vi "Generate Z stage Position Aarray.vi"(7 "#rep1":i32, 8 "#rep2":u16, 9 "thickness2":dbl, 10 "Start Z":dbl format="%#_13g", 11 "thickness1":dbl) -> (3 "Array":dbl[](array[numeric]))   [LabVIEW 2018]
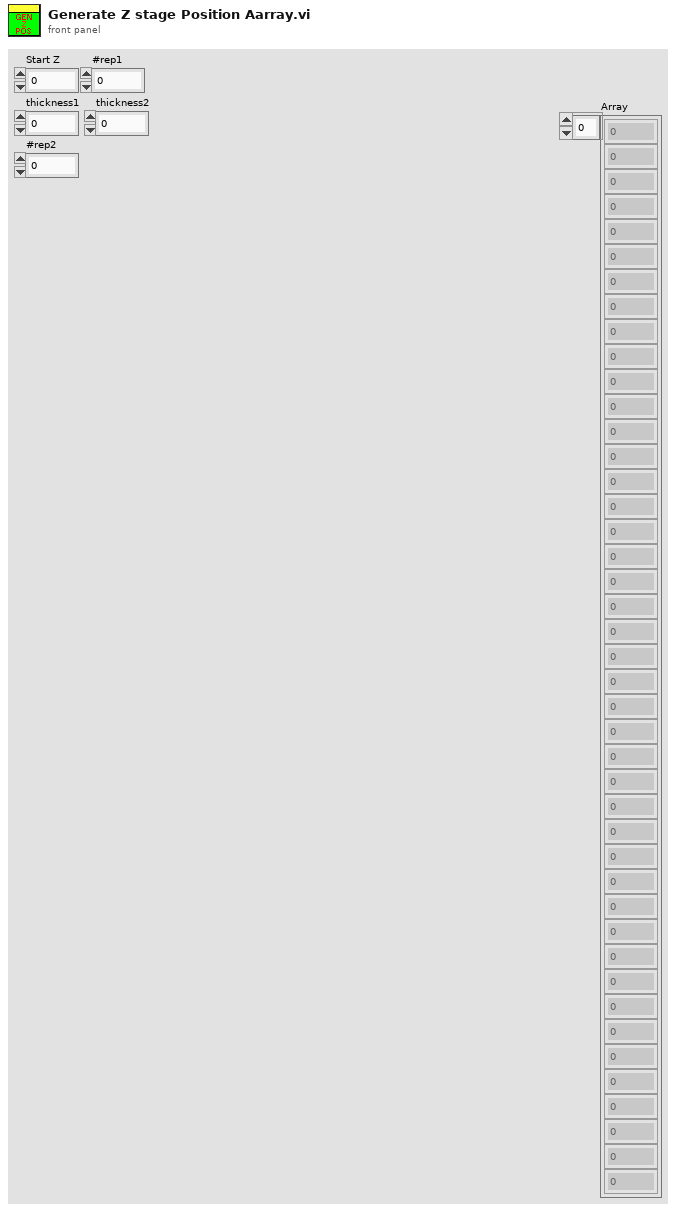
[diagram p1: front panel]
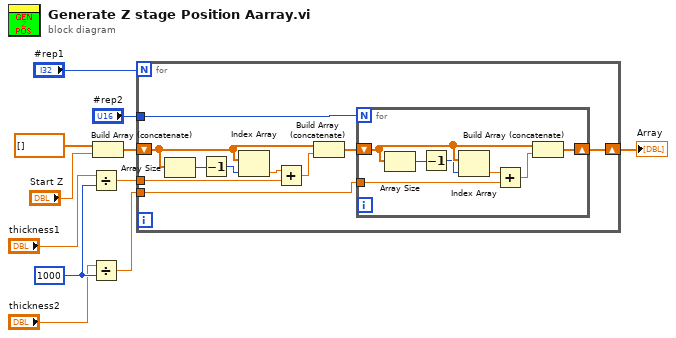
[diagram p0: block diagram]
diagram:
  w11 = 1000
  n1 = Divide(x="thickness1", y=w11) -> (x/y=w9:dbl)
  n2 = Divide(x="thickness2", y=w11) -> (x/y=w10:dbl)
  n3 = Build Array (concatenate)(dbl[] [] ("element"), "Start Z") -> (w7:dbl[])
  n4 = for {
    N: "#rep1" -> [_]
    shift-right: [w18] -> w6
    shift-left: w7 -> [w15]
    tunnel: w9 -> [w16]
    tunnel: w10 -> [w19]
    tunnel: "#rep2" -> [w21]
    n5 = Array Size(array=w15) -> (size(s)=w13:i32)
    n6 = Decrement(x=w13) -> (x-1=w12:i32)
    n7 = Index Array(array=w15, index=w12) -> (element=w17:dbl)
    n8 = Add(x=w17, y=w16) -> (x+y=w14:dbl)
    n9 = Build Array (concatenate)(w15, w14) -> (w20:dbl[])
    n10 = for {
      N: w21 -> [_]
      tunnel: w19 -> [w25]
      shift-right: [w28] -> w18
      shift-left: w20 -> [w27]
      n11 = Array Size(array=w27) -> (size(s)=w22:i32)
      n12 = Decrement(x=w22) -> (x-1=w23:i32)
      n13 = Index Array(array=w27, index=w23) -> (element=w26:dbl)
      n14 = Add(x=w26, y=w25) -> (x+y=w24:dbl)
      n15 = Build Array (concatenate)(w27, w24) -> (w28:dbl[])
    }
  }
  "Array" <- w6
